vi "destroyObject.vi"(0 "HGF_Factory":refnum<class "HGF_Factory.lvclass">, 5 "error in (no error)":errorcluster) -> (19 "error out":errorcluster)   [LabVIEW 2014, in "HGF_BaseClasses.lvlib" / "HGF_Factory.lvclass"]
uses:
  HGF_Factory.lvclass
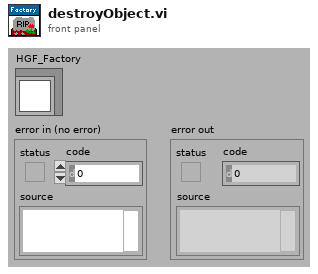
[diagram p1: front panel]
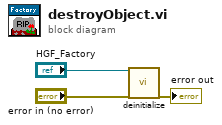
[diagram p0: block diagram]
diagram:
  n1 = call-dynamic "deinitialize.vi"("HGF_Factory"="HGF_Factory", "error in (no error)"="error in (no error)") -> ("error out"=→"error out":errorcluster)  [unwired: 17 in]
